vi "TellActor.vi"(9 "ActorAlias":string, 10 "Message":refnum<class "Message.lvclass">, 11 "Actor":refnum<class "Actor.lvclass">) -> (3 "Actor":refnum<class "Actor.lvclass">)   [LabVIEW 2020, in "jettl.lvlib"]
uses:
  jettl.lvlib
  ActorRelation.ctl
  Actor/Actor.lvclass
  Message/Message.lvclass
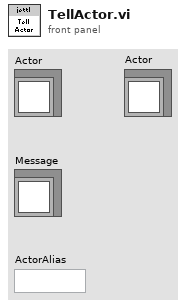
[diagram p1: front panel]
types:
  T1 = typedef "jettl.lvlib/Actor.ctl" = cluster{"Messages":T2, "Alias":string, "Transport":refnum<user-event>, "Address":refnum<event-registration>, "VIRef":refnum<vi>, "ActorType":T4}
  T2 = typedef "jettl.lvlib/Messages.ctl" = cluster{"Listen":T3, "Tell":T3, "TellSelf":T3, "TellActor":T3}
  T3 = typedef "jettl.lvlib/MessageSet.ctl" = set{refnum<class "Message.lvclass">}
  T4 = typedef "jettl.lvlib/ActorType.ctl" = enum16{"Mediator", "Component"}
  T5 = typedef "jettl.lvlib/BaseActor.ctl" = cluster{"ActorLifetime":T6, "SelfActor":T1, "ActorMap":T7}
  T6 = typedef "jettl.lvlib/ActorLifetime.ctl" = enum16{"Init", "Spawn", "Setup", "Teardown Before Running", "Running", "Stop Called", "Stopping With Children", "Stopping Without Children", "Teardown After Running", "Stopped"}
  T7 = typedef "jettl.lvlib/ActorMap.ctl" = map{string, T1}
  T8 = typedef "jettl.lvlib/ActorRelation.ctl" = enum16{"Self", "Actor"}
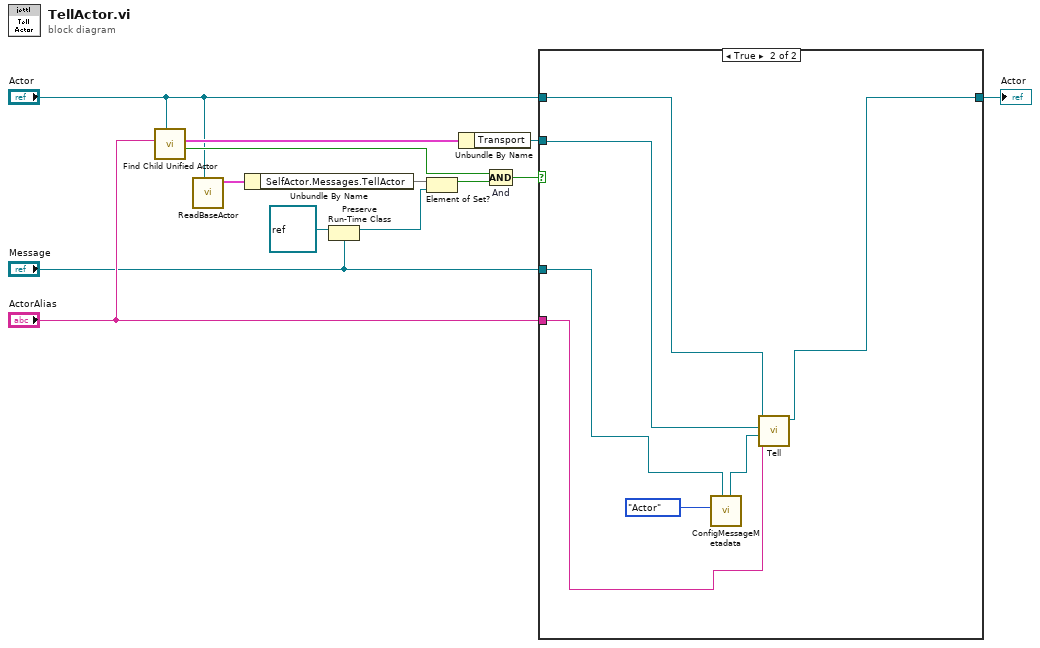
[diagram p0: block diagram]
diagram:
  n1 = call "Find Child Unified Actor.vi"("Actor in"="Actor", "Unified Actor Alias"="ActorAlias") -> ("Found"=w7:bool, "Child Unified Actor"=w11:T1)  [unwired: 8 in]
  n2 = call-dynamic "ReadBaseActor.vi"("Actor in"="Actor") -> ("BaseActor"=w4:T5)  [unwired: 10 in]
  n3 = Unbundle By Name(w4) -> ("SelfActor.Messages.TellActor"=w8:T3)
  n4 = Preserve Run-Time Class(object in=refnum<class> refnum, 2:"Message") -> (object out=w1:refnum<class "Message.lvclass">)  [unwired: 1 in, 1 out]
  n5 = Element of Set?(10:w1, 11:w8) -> (3:w9:bool)
  n6 = Unbundle By Name(w11) -> ("Transport"=w10:refnum<user-event>)
  n7 = Compound Arithmetic op=AND "And"(w7, w9) -> (w6:bool)
  n8 = case shown="True" w6 {
    tunnel: "Actor" -> [w14 w15]
    tunnel: [w14 w17] -> w12
    tunnel: "ActorAlias" -> [_ w16]
    tunnel: w10 -> [_ w18]
    tunnel: "Message" -> [_ w19]
    frame False {
    }
    frame True {
      n9 = call-dynamic "ConfigMessageMetadata.vi"("Message"=w19, "ActorRelation"=ActorRelation."Actor") -> ("Message"=w21:refnum<class "Message.lvclass">)  [unwired: 9 in]
      n10 = call "Tell.vi"("ActorAlias"=w16, "Message"=w21, "Transport"=w18, "Actor"=w15) -> ("Actor"=w17:refnum<class "Actor.lvclass">)  [unwired: 7 in]
    }
  }
  "Actor" <- w12
